vi "Global 12.vi"() -> ()   [LabVIEW 2015]
panel:
  out "Sine 2":dynamicdata(graph) caption="Sine"
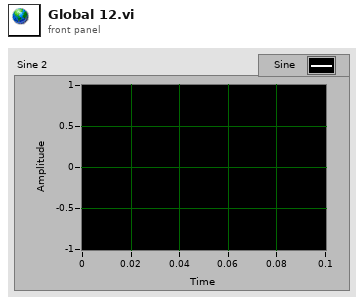
[diagram p1: front panel]
diagram:
